vi "Write Peaks buffer.vi"(8 "error in (no error)":errorcluster, 10 "Peaks buffer":dbl[][](array[numeric]), 11 "Micron Optics Driver in":refnum<class "Micron Optics Driver.lvclass">) -> (0 "error out":errorcluster, 3 "Micron Optics Driver out":refnum<class "Micron Optics Driver.lvclass">)   [LabVIEW 2016, in "Micron Optics Driver.lvclass"]
uses:
  Micron Optics Driver.lvclass
  Micron Optics Driver.lvclass/Micron Optics Driver.ctl
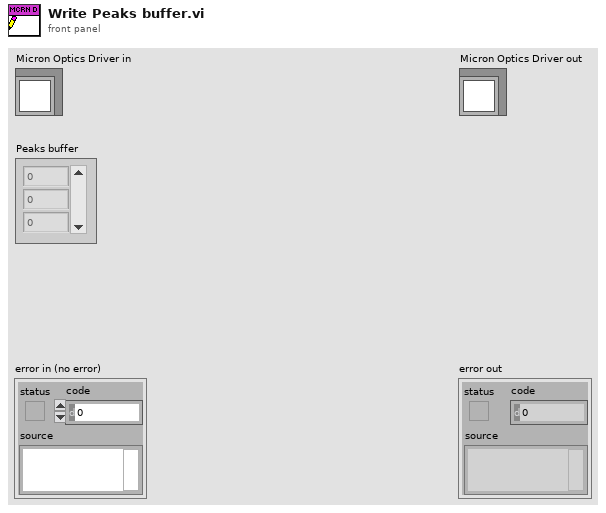
[diagram p1: front panel]
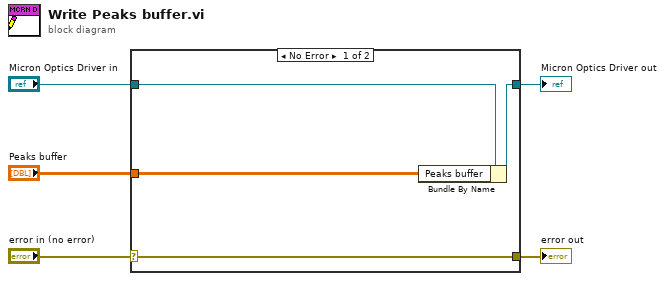
[diagram p0: block diagram]
diagram:
  n1 = case shown="No Error" "error in (no error)" {
    selector: "error in (no error)" -> [w9 w10]
    tunnel: [w9 w10] -> w4
    tunnel: [w7 w11] -> w2
    tunnel: "Micron Optics Driver in" -> [w8 w11]
    tunnel: "Peaks buffer" -> [w6 _]
    frame No Error {
      n2 = Bundle By Name(cluster=w8, "Peaks buffer"=w6) -> (w7:refnum<class "Micron Optics Driver.lvclass">)
    }
    frame Error {
    }
  }
  "error out" <- w4
  "Micron Optics Driver out" <- w2
